vi "Position Delete Waypoint Button.vi"(8 "error in (no error)":errorcluster, 10 "Previous Button Refnum":refnum<vi>, 11 "Shutdon Button":refnum<vi>) -> (0 "error out":errorcluster)   [LabVIEW 2014]
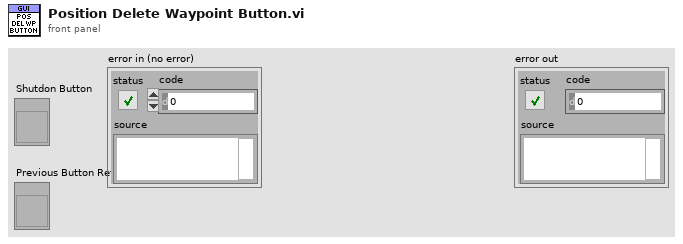
[diagram p1: front panel]
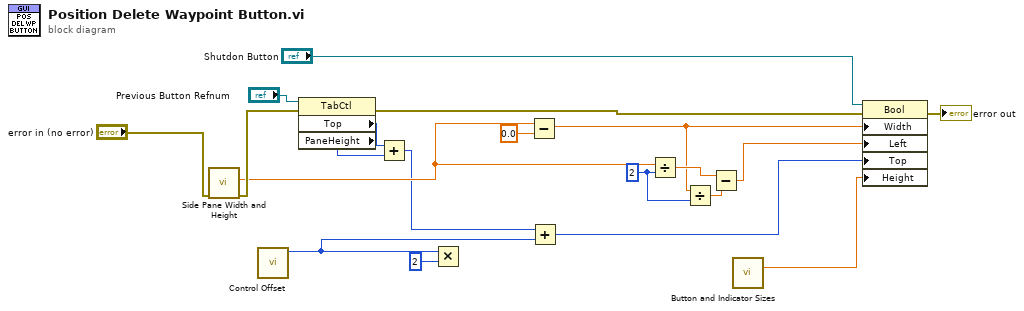
[diagram p0: block diagram]
diagram:
  w13 = u32 2 ("y")
  n1 = call "Side Pane Width and Height.vi"("error in (no error)"="error in (no error)") -> ("error out"=w7:errorcluster, "Width"=w6:dbl)  [unwired: 8 in, 1 out]
  n2 = call "Control Offset.vi"() -> ("Offset From Tab Edge in (px)"=w16:i32)  [unwired: 11 in]
  n3 = property class="TabCtl"(reference="Previous Button Refnum", error in=w7) -> (error out=w17:errorcluster, "Top"=w5:i32, "PaneHeight"=w4:u32)  [unwired: 1 out]
  n4 = Add(x=w5, y=w4) -> (x+y=w3:u32)
  n5 = Multiply(x=w16, y=2) -> ()  [unwired: 1 out]
  n6 = Subtract(x=w6, y=0.0) -> (x-y=w12:dbl)
  n7 = Add(x=w3, y=w16) -> (x+y=w15:u32)
  n8 = Divide(x=w6, y=w13) -> (x/y=w14:dbl)
  n9 = Divide(x=w12, y=w13) -> (x/y=w11:dbl)
  n10 = Subtract(x=w14, y=w11) -> (x-y=w10:dbl)
  n11 = call "Button and Indicator Sizes.vi"() -> ("Button Height"=w2:dbl)  [unwired: 11 in, 4 out]
  n12 = property class="Bool"(reference="Shutdon Button", error in=w17, "Width"=w12, "Left"=w10, "Top"=w15, "Height"=w2) -> (error out=→"error out":errorcluster)  [unwired: 1 out]
